vi "Лабораторная №1 Задание 3_3.vi"() -> ()   [LabVIEW 2017]
panel:
  in  "Frequency":dbl
  in  "stop":bool
  in  "Knob":dbl(knob) scale=0.0..10.0
  out "Waveform Graph":dynamicdata(graph)
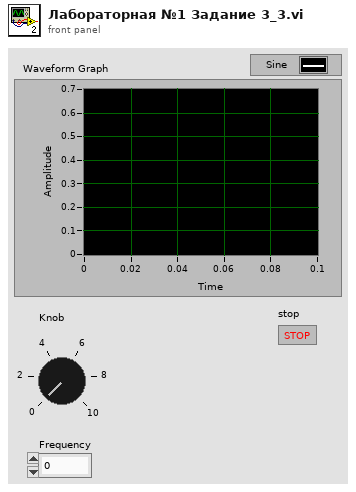
[diagram p1: front panel]
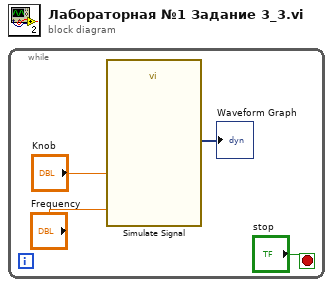
[diagram p0: block diagram]
diagram:
  n1 = while {
    stop <- "stop" stop-if-true
    n2 = call "Simulate Signal"("Frequency"="Frequency", "Amplitude"="Knob") -> ("Sine"=→"Waveform Graph":dynamicdata)  [unwired: 12 in, 1 out]
  }
